vi "FTW-Package-Multipart-Initialize.vi"(0 "FTW Message":refnum<class "FTW-Package.lvclass">, 5 "Message Parts":string[](array[string]), 11 "error in":errorcluster) -> (4 "FTW Message out":refnum<class "FTW-Package.lvclass">, 15 "error out":errorcluster)   [LabVIEW 2013, in "FTW-Package.lvclass"]
uses:
  FTW-Package.lvclass
  FTW-Package.lvclass/FTW-Package.ctl
panel:
  # "Inputs"
  # "Outputs"
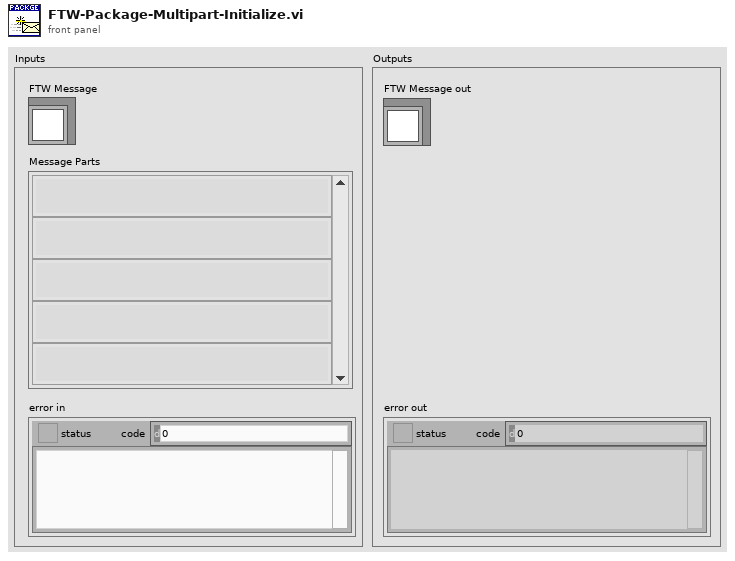
[diagram p1: front panel]
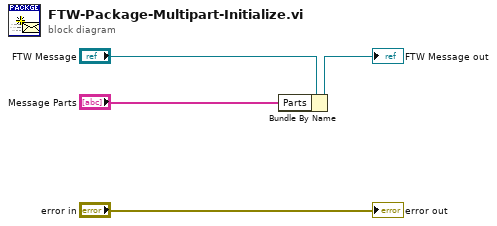
[diagram p0: block diagram]
diagram:
  n1 = Bundle By Name(cluster="FTW Message", "Parts"="Message Parts") -> (→"FTW Message out":refnum<class "FTW-Package.lvclass">)
  "error out" <- "error in"
